vi "Release.vi"(8 "error in (no error)":errorcluster, 11 "Execution in":refnum<class "Execution.lvclass">) -> (0 "error out":errorcluster)   [LabVIEW 2020, in "TSnax.lvlib" / "Execution.lvclass"]
uses:
  Execution.lvclass
  Execution.lvclass/Execution.ctl
  PropertyObject/PropertyObject.lvclass/PropertyObject.ctl
  PropertyObject/PropertyObject Ref.vi
  SequenceFile/SequenceFile.lvclass
  C:/dev/illuminated-g/tsnax/TSnax/PropertyObject/PropertyObject.lvclass
  PropertyObject/PropertyObject.lvclass
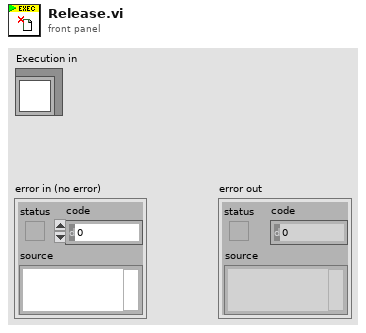
[diagram p1: front panel]
types:
  T1 = typedef "TSnax.lvlib/Execution.lvclass/Ref Data.ctl" = cluster{"Parameters":refnum<class "PropertyObject.lvclass">, "Client Sequence":refnum<class "SequenceFile.lvclass">, "Process Model":refnum<class "SequenceFile.lvclass">, "Entry Sequence":string, "Execution":refnum<k7>, "Report":refnum<class "Report.lvclass">, "Options":T2}
  T2 = typedef "TSnax.lvlib/Execution.lvclass/Execution Options.ctl" = cluster{"Use Default Model":bool, "Release Related References":bool}
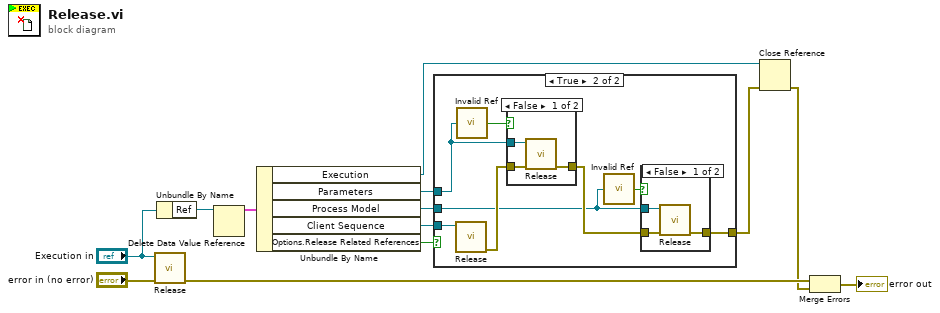
[diagram p0: block diagram]
diagram:
  n1 = call-parent "Release.vi"("error in (no error)"="error in (no error)", "PropertyObject in"="Execution in") -> ("error out"=w3:errorcluster)  [unwired: 9 in]
  n2 = Unbundle By Name("Execution in") -> ("Ref"=w11:refnum<data-value>)
  n3 = Delete Data Value Reference(data value reference=w11) -> (data value=w10:T1)  [unwired: 1 in, 1 out]
  n4 = Unbundle By Name(w10) -> ("Execution"=w5:refnum<k7>, "Parameters"=w6:refnum<class "PropertyObject.lvclass">, "Process Model"=w7:refnum<class "SequenceFile.lvclass">, "Client Sequence"=w8:refnum<class "SequenceFile.lvclass">, "Options.Release Related References"=w9:bool)
  n5 = case shown="True" w9 {
    tunnel: w8 -> [_ w21]
    tunnel: w7 -> [_ w15]
    tunnel: w6 -> [_ w19]
    tunnel: [_ w14] -> w4
    frame False {
    }
    frame True {
      n6 = call-dynamic "Release.vi"("SequenceFile in"=w21) -> ("error out"=w18:errorcluster)  [unwired: 10 in]
      n7 = call "Invalid Ref.vi"("PropertyObject"=w19) -> ("Not a Valid Ref?"=w20:bool)
      n8 = case shown="False" w20 {
        tunnel: w19 -> [w28 _]
        tunnel: [w27 w29] -> w16
        tunnel: w18 -> [w26 w29]
        frame False {
          n9 = call-dynamic "Release.vi"("error in (no error)"=w26, "PropertyObject in"=w28) -> ("error out"=w27:errorcluster)  [unwired: 9 in]
        }
        frame True {
        }
      }
      n10 = call "Invalid Ref.vi"("PropertyObject"=w15) -> ("Not a Valid Ref?"=w17:bool)
      n11 = case shown="False" w17 {
        tunnel: w15 -> [w24 _]
        tunnel: [w23 w25] -> w14
        tunnel: w16 -> [w22 w25]
        frame False {
          n12 = call-dynamic "Release.vi"("error in (no error)"=w22, "SequenceFile in"=w24) -> ("error out"=w23:errorcluster)  [unwired: 9 in]
        }
        frame True {
        }
      }
    }
  }
  n13 = Close Reference(reference=w5, error in (no error)=w4) -> (error out=w2:errorcluster)
  n14 = Merge Errors(w3, w2) -> (→"error out":errorcluster)
